vi "h5_write_xwav.vi"(7 "object name":string, 8 "error in":errorcluster, 10 "xwave":T1={"attributes"=variant, "X"={"start"=0.0, "delta"=0.0, "units"="index", "dim"="au"}, "Y"={"data"=[], "units"="au"}}, 11 "h5 ref in":T2 format="%.0x") -> (0 "error out":errorcluster, 2 "dup xwave":T1={"attributes"=variant, "X"={"start"=0.0, "delta"=0.0, "units"="index", "dim"="au"}, "Y"={"data"=[], "units"="au"}}, 3 "dup h5 ref":T2 format="%.0x")   [LabVIEW 2015]
uses:
  <vilib>/addons/h5labview2/base/hid_t.ctl
  xwave/xwav.ctl
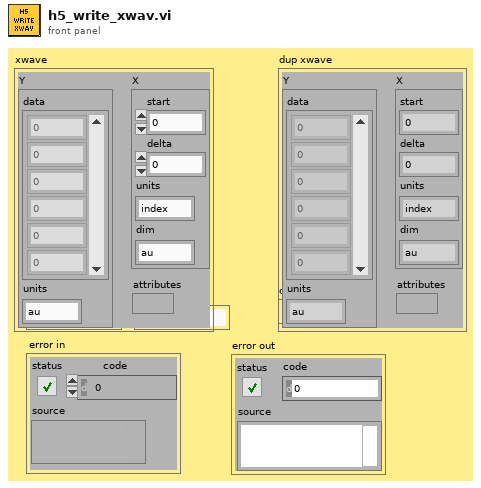
[diagram p1: front panel]
types:
  T1 = typedef "xwav.ctl" = cluster{"attributes":variant, "X":cluster{"start":dbl, "delta":dbl, "units":string, "dim":string}, "Y":cluster{"data":dbl[], "units":string}}
  T2 = typedef "hid_t.ctl" = i32
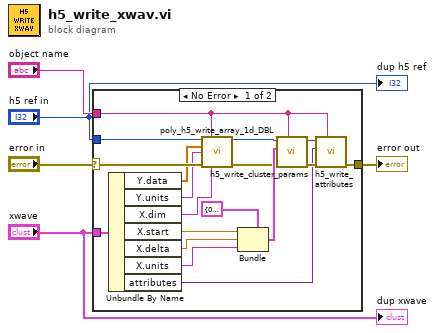
[diagram p0: block diagram]
diagram:
  n1 = case shown="No Error" "error in" {
    selector: "error in" -> [w19 w24]
    tunnel: [w20 w24] -> w5
    tunnel: "h5 ref in" -> [w18 _]
    tunnel: "xwave" -> [w23 _]
    tunnel: "object name" -> [w10 _]
    frame No Error {
      n2 = Unbundle By Name(w23) -> ("Y.data"=w15:dbl[], "Y.units"=w14:string, "X.dim"=w13:string, "X.start"=w12:dbl, "X.delta"=w11:dbl, "X.units"=w9:string, "attributes"=w6:variant)
      n3 = call "poly_h5_write_array_1d_DBL.vi"("h5 dir ref"=w18, "dataset name"=w10, "array"=w15, "units (au)"=w14, "error in (no error)"=w19, "dim (index)"=w13) -> ("h5 obj ref"=w17:i32, "error out"=w16:errorcluster)  [unwired: 8 in]
      n4 = Bundle(cluster=cluster{"x0":dbl, "dx":dbl, "x units":string} {"x0"=0.0, "dx"=0.0, "x units"=""} ("xwave"), "x0"=w12, "dx"=w11, "x units"=w9) -> (w21:cluster{"x0":dbl, "dx":dbl, "x units":string})
      n5 = call "h5_write_cluster_params.vi"("object name"=w10, "error in (no error)"=w16, "cluster"=w21, "h5 dir/obj ref"=w17) -> ("error out"=w7:errorcluster, "h5 dir/obj ref"=w8:T2)  [unwired: 6 in]
      n6 = call "h5_write_attributes.vi"("object name"=w10, "error in"=w7, "attributes"=w6, "h5 ref"=w8) -> ("error out"=w20:errorcluster)  [unwired: 6 in, 1 out]
    }
    frame Error {
    }
  }
  "error out" <- w5
  "dup h5 ref" <- "h5 ref in"
  "dup xwave" <- "xwave"
